vi "AM Elapsed Time.vi"(11 "AM Refs in":T1 {"PS Measure Plan" items=["Pretreatment settings (PS)", "Linear Sweep Voltammetry (LSV)", "Differential Pulse Voltammetry (DPV)", "Cyclic Voltammetry (CV)", "Chronoamperometry (CA)", "Chronopotentiometry (CP)", "El Imp Spectroscopy (EIS)"]; "System Preset"."Test Configuration"."SP List" format="%#.1g"}) -> (1 "Time has Elapsed":bool, 2 "Start Elapsed Time":dbl caption="Elapsed Time (s)", 3 "AM Refs out":T1 {"PS Measure Plan" items=["Pretreatment settings (PS)", "Linear Sweep Voltammetry (LSV)", "Differential Pulse Voltammetry (DPV)", "Cyclic Voltammetry (CV)", "Chronoamperometry (CA)", "Chronopotentiometry (CP)", "El Imp Spectroscopy (EIS)"]; "System Preset"."Test Configuration"."SP List" format="%#.1g"}, 4 "Elapsed Time (s)":dbl)   [LabVIEW 2020, in "Test Driver.lvlib"]
uses:
  Test Driver.lvlib
  Test Driver Configuration.ctl
  support/Message Queue/Message Cluster.ctl
  System Preset.ctl
  Test Type.ctl
  support/Message Queue/Message Queue.lvlib
panel:
  # "X"
  # "Y"
  # "Cycles"
  # "Point Delay"
  # "Up"
  # "Down"
  # "Z Axes"
  # "#C"
  # "In"
  # "Out"
  # "Cleaning [sec]"
  # "X"
  # "Y"
  # "Cycles"
  # "Point Delay"
  # "Up"
  # "Down"
  # "Z Axes"
  # "#C"
  # "In"
  # "Out"
  # "Cleaning [sec]"
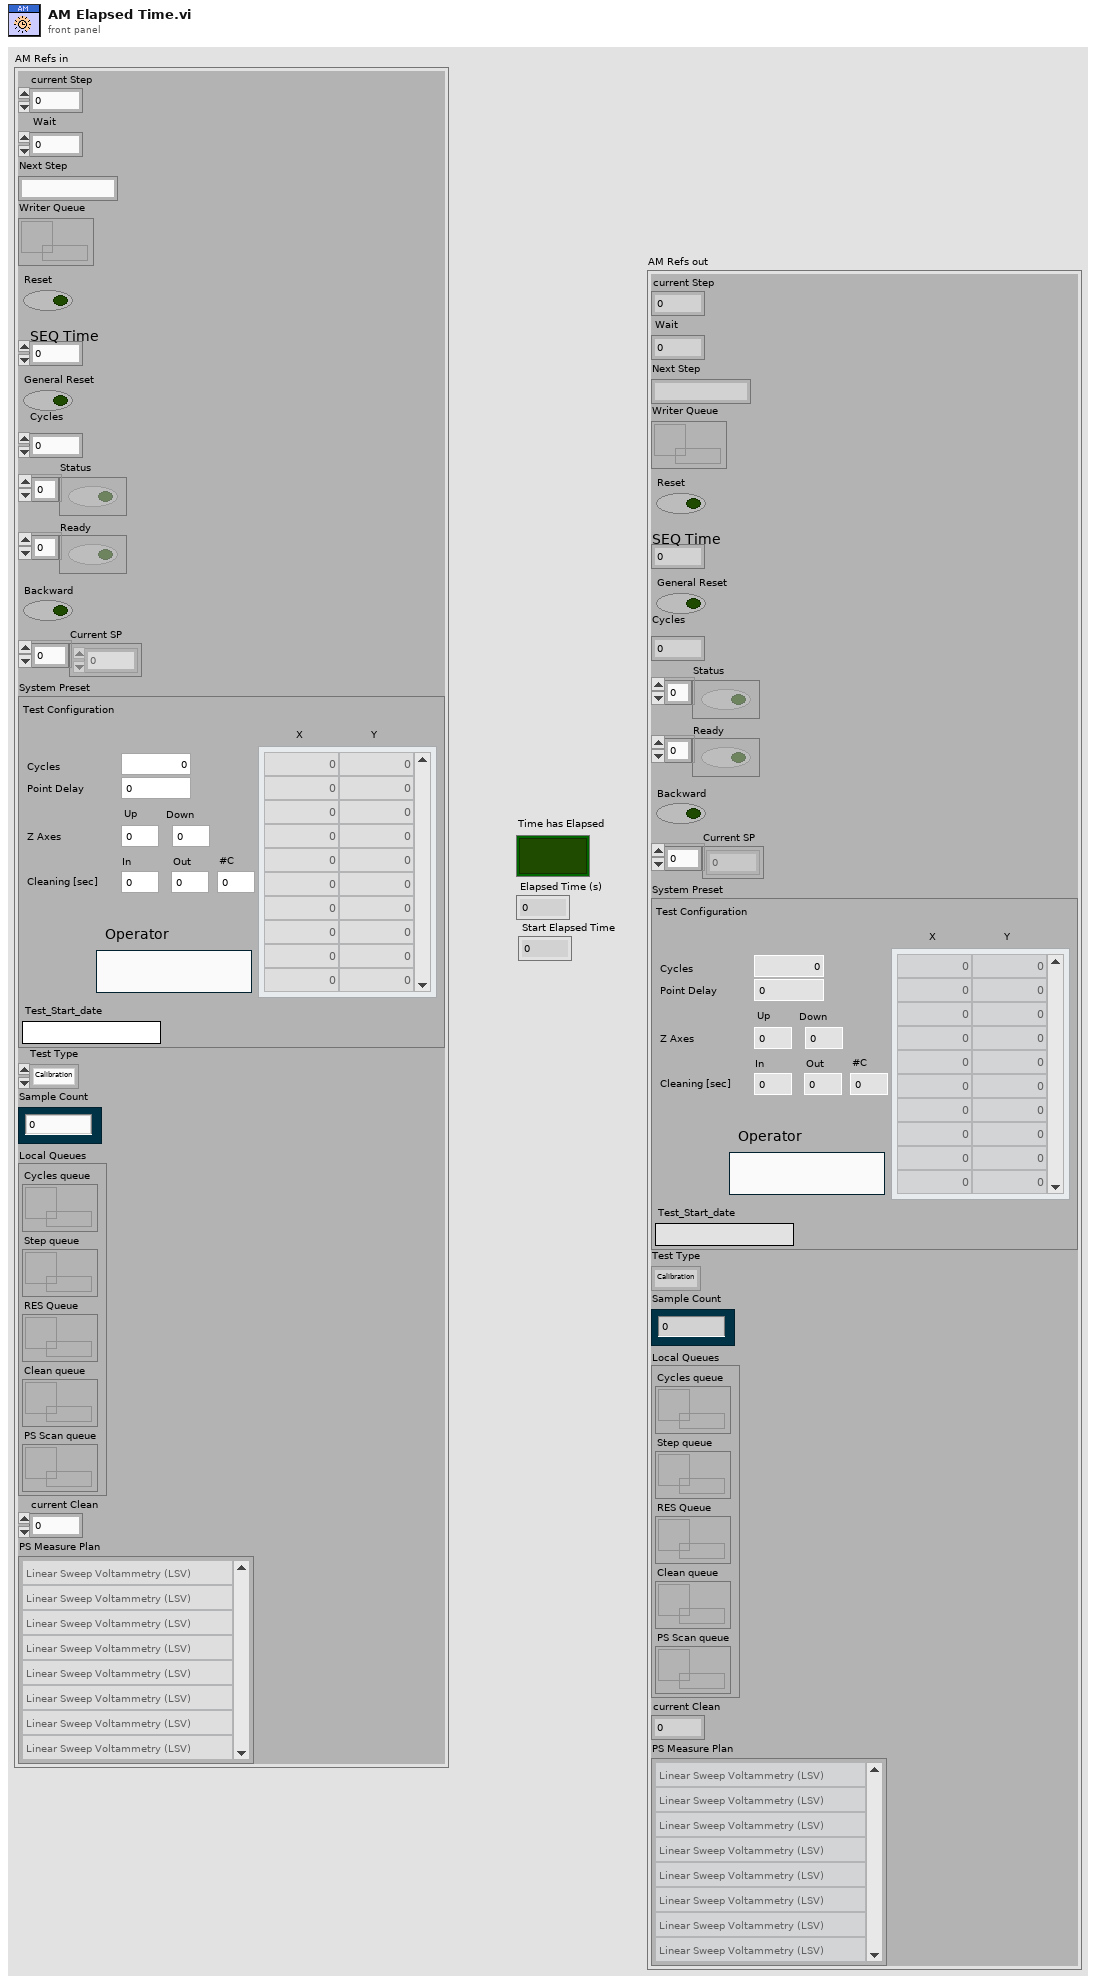
[diagram p1: front panel]
types:
  T1 = typedef "Test Driver.lvlib/Test Driver Configuration.ctl" = cluster{"current Step":i32, "Wait":dbl, "Next Step":string, "Writer Queue":refnum<queue>, "Reset":bool, "SEQ Time":i32, "General Reset":bool, "Cycles":i32, "Status":bool[], "Ready":bool[], "Backward":bool, "Current SP":dbl[], "System Preset":T2, "Test Type":T3, "Sample Count":i32, "Local Queues":cluster{"Cycles queue":refnum<queue>, "Step queue":refnum<queue>, "RES Queue":refnum<queue>, "Clean queue":refnum<queue>, "PS Scan queue":refnum<queue>}, "current Clean":i32, "PS Measure Plan":u16[]}
  T2 = typedef "System Preset.ctl" = cluster{"Test Configuration":cluster{"Cycles":i32, "Z Up":dbl, "SP List":dbl[][], "Operator":string, "Point Delay":i32, "Z Up 2":dbl, "Cleaning In":dbl, "Cleaning Out":dbl, "Cleaning Cycles":i32}, "Test_Start_date":string}
  T3 = typedef "Test Driver.lvlib/Test Type.ctl" = enum16{"Calibration", "Test"}
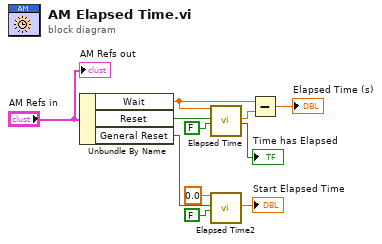
[diagram p0: block diagram]
diagram:
  n1 = Unbundle By Name("AM Refs in") -> ("Wait"=w7:dbl, "Reset"=w9:bool, "General Reset"=w3:bool)
  n2 = call "Elapsed Time"("Time Target (s)"=w7, "Reset"=w9, "Auto Reset"=FALSE) -> ("Elapsed Time (s)"=w6:dbl, "Time has Elapsed"=→"Time has Elapsed":bool)  [unwired: 9 in, 6 out]
  n3 = call "Elapsed Time2"("Time Target (s)"=0.0, "Reset"=w3, "Auto Reset"=FALSE) -> ("Elapsed Time (s)"=→"Start Elapsed Time":dbl)  [unwired: 9 in, 7 out]
  n4 = Subtract(x=w7, y=w6) -> (x-y=→"Elapsed Time (s)":dbl)
  "AM Refs out" <- "AM Refs in"
